vi "0 less than x less than 3.5.vi"(1 "x":fxp<+/-,20,5> format="%.17g") -> (0 "coerced x":fxp<+/-,20,5> format="%.17g")   [LabVIEW 2009]
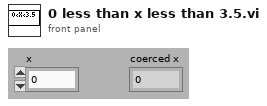
[diagram p1: front panel]
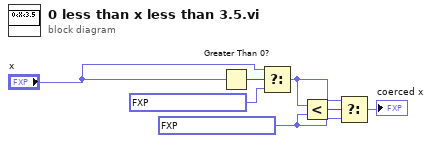
[diagram p0: block diagram]
diagram:
  w6 = fxp<+/-,20,5> 3.5 ("y")
  n1 = Greater Than 0?(x="x") -> (x > 0?=w4:bool)
  n2 = Select(t="x", s=w4, f=fxp<+/-,20,5> 0.0) -> (s? t:f=w3:fxp<+/-,20,5>)
  n3 = Less?(x=w3, y=w6) -> (x < y?=w5:bool)
  n4 = Select(t=w3, s=w5, f=w6) -> (s? t:f=→"coerced x":fxp<+/-,20,5>)
